vi "Test_HelloWorld_Internationalization.vi"() -> (0 "Array of Error Description":T1)   [LabVIEW 2019]
uses:
  gRPC_ATS/TestUtility/utility.llb/array of error description.ctl
  gRPC_ATS/TestUtility/utility.llb/error description.ctl
  gRPC_ATS/TestUtility/utility.llb/error type.ctl
  examples/helloworld/helloworld_client/RPC Messages/helloworld_HelloReply.ctl
  examples/helloworld/helloworld_client/RPC Messages/helloworld_HelloRequest.ctl
  examples/helloworld/helloworld_client/helloworld_client.lvlib
panel:
  out "Pass":bool
  in  "Client VI Path":path=path "../../examples/helloworld/helloworld_client/Run greeter_client.vi"
  in  "Server VI path":path=path "../../examples/helloworld/helloworld_server/Run greeter_server.vi"
  in  "error in (no error)":errorcluster
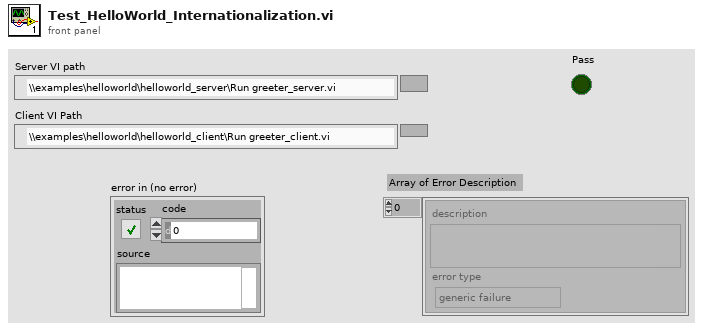
[diagram p1: front panel]
types:
  T1 = typedef "array of error description.ctl" = T2[]
  T2 = typedef "error description.ctl" = cluster{"description":string, "error type":T3}
  T3 = typedef "error type.ctl" = enum32{"generic failure", "boundary case", "precision", "expected error"}
  T4 = typedef "helloworld_client.lvlib/helloworld_HelloRequest.ctl" = cluster{"name":string}
  T5 = typedef "helloworld_client.lvlib/helloworld_HelloReply.ctl" = cluster{"message":string}
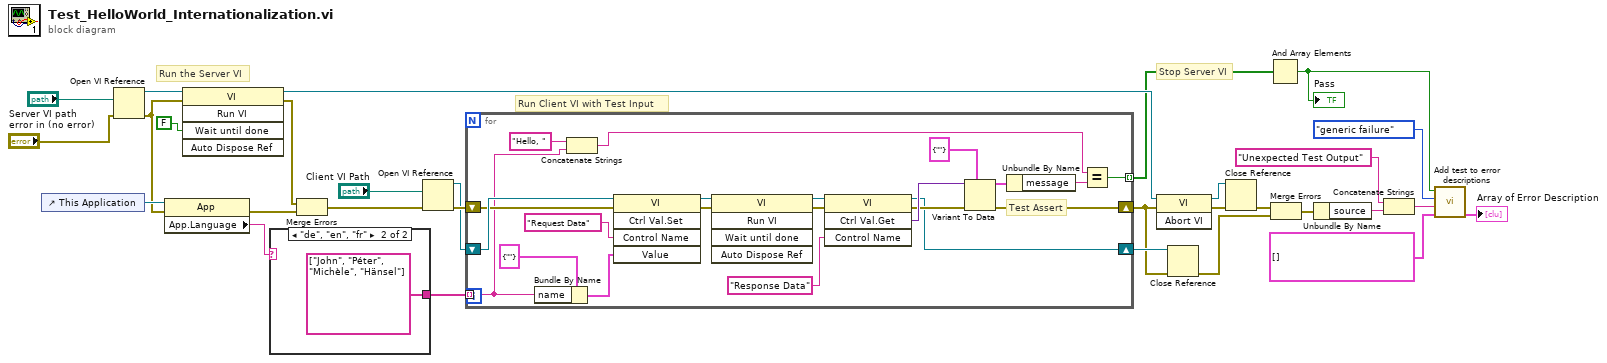
[diagram p0: block diagram]
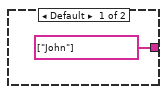
[diagram p2: hidden frame]
diagram:
  # "Run the Server VI"
  # "Run Client VI with Test Input"
  # "Stop Server VI"
  n1 = control-ref of="This Application"() -> (w5:refnum<vi>)
  n2 = Open VI Reference(vi path="Server VI path", error in (no error)="error in (no error)") -> (vi reference=w8:refnum<vi>, error out=w2:errorcluster)  [unwired: 4 in]
  n3 = property class="App"(reference=w5, error in=w2) -> (error out=w3:errorcluster, "App.Language"=w4:string)  [unwired: 1 out]
  n4 = invoke class="VI" method="Run VI"(reference=w8, error in=w2, "Wait until done"=FALSE ("Wait Until Done")) -> (reference out=w22:refnum<vi>, error out=w6:errorcluster)  [unwired: 2 in, 3 out]
  n5 = case shown="\"de\", \"en\", \"fr\"" w4 {
    tunnel: [string[] ["John"] string[] ["John", "Péter", "Michèle", "Hänsel"]] -> w1
    frame Default {
    }
    frame "de", "en", "fr" {
    }
  }
  n6 = Merge Errors(w6, w3) -> (w15:errorcluster)
  n7 = Open VI Reference(vi path="Client VI Path", error in (no error)=w15) -> (vi reference=w13:refnum<vi>, error out=w14:errorcluster)  [unwired: 4 in]
  n8 = for {
    tunnel: [w34] -> w21 mode=indexing
    shift-right: [w53] -> w12
    shift-left: w14 -> [w39]
    shift-right: [w40] -> w17
    shift-left: w13 -> [w48]
    tunnel: w1 -> [w33] mode=indexing
    # "Test Assert"
    n9 = Bundle By Name(cluster=T4 {"name"=""} ("helloworld_HelloRequest"), "name"=w33) -> (w35:T4)
    n10 = Concatenate Strings("Hello, " ("string"), w33) -> (w36:string)
    n11 = invoke class="VI" method="Ctrl Val.Set"(reference=w48, error in=w39, "Control Name"="Request Data" ("Control Label"), "Value"=w35) -> (reference out=w47:refnum<vi>, error out=w38:errorcluster)  [unwired: 1 in, 3 out]
    n12 = invoke class="VI" method="Run VI"(reference=w47, error in=w38) -> (reference out=w45:refnum<vi>, error out=w44:errorcluster)  [unwired: 3 in, 3 out]
    n13 = invoke class="VI" method="Ctrl Val.Get"(reference=w45, error in=w44, "Control Name"="Response Data" ("Control Label")) -> (reference out=w40:refnum<vi>, error out=w41:errorcluster, "Get Control Value Variant"=w42:variant)  [unwired: 1 in, 1 out]
    n14 = Variant To Data(error in=w41, type=T5 {"message"=""} ("Response Data"), Variant=w42) -> (data=w50:T5, error out=w53:errorcluster)
    n15 = Unbundle By Name(w50) -> ("message"=w49:string)
    n16 = Equal?(x=w36, y=w49) -> (x = y?=w34:bool)
  }
  n17 = invoke class="VI" method="Abort VI"(reference=w22, error in=w12) -> (reference out=w23:refnum<vi>, error out=w24:errorcluster)  [unwired: 1 in, 1 out]
  n18 = Close Reference(reference=w17, error in (no error)=w12) -> (error out=w19:errorcluster)
  n19 = Close Reference(reference=w23, error in (no error)=w24) -> (error out=w20:errorcluster)
  n20 = And Array Elements(Boolean array=w21) -> (logical AND=w11:bool)
  "Pass" <- w11
  n21 = Merge Errors(w20, w19) -> (w18:errorcluster)
  n22 = Unbundle By Name(w18) -> ("source"=w26:string)
  n23 = Concatenate Strings("Unexpected Test Output" ("string"), w26) -> (w27:string)
  n24 = call "Add test to error descriptions.vi"("error descriptions in"=T1 [], "error string"=w27, "error type"=error_type."generic failure", "pass"=w11) -> ("error description out"=→"Array of Error Description":T1)  [unwired: 3 in]
